vi "(Sub_VI)_CustomPID_BIST.vi"(0 "Process Value":dbl=0.0005 format="%_9g", 1 "Max Out":dbl=0.0005, 2 "Ed_in":dbl, 3 "Min Out":dbl=0.0005, 5 "Set Point":dbl=0.0005 format="%_9g", 7 "Ei_in":dbl, 9 "Kp":dbl, 11 "Kd":dbl, 12 "Ki":dbl) -> (4 "DutyCycle":dbl, 6 "Cp":dbl, 8 "Ei_out":dbl, 10 "Ci":dbl, 13 "Ed_out":dbl, 15 "Cd":dbl)   [LabVIEW 2019]
doc: "The initial value of shift registers (1) and (2) should be left open. If we add zero inside this sub-vi then the integral and the dirivitive of the error is calculated wrong"
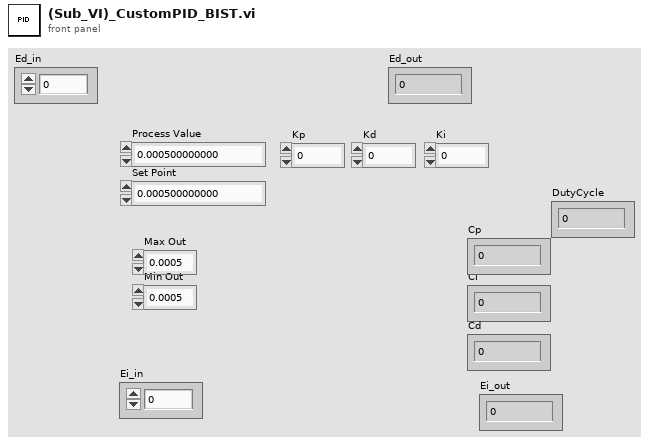
[diagram p1: front panel]
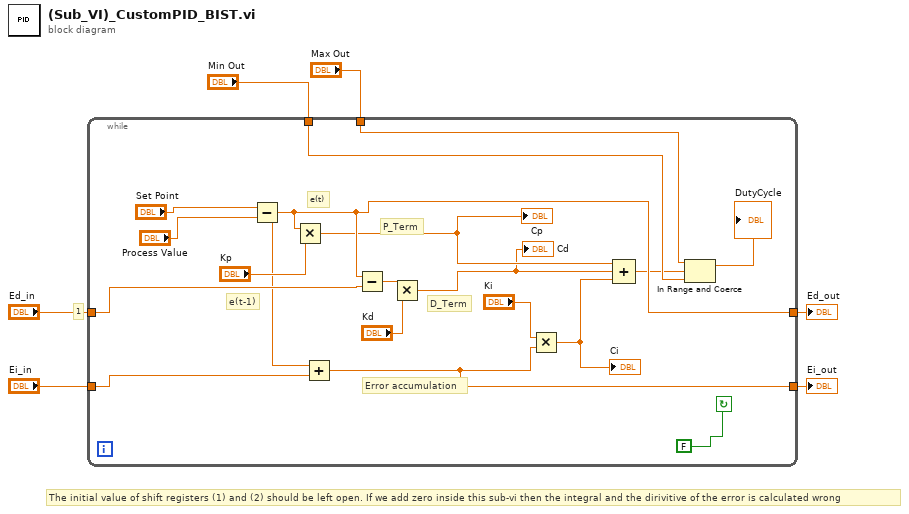
[diagram p0: block diagram]
diagram:
  # "1"
  # "The initial value of shift registers (1) and (2) should be left open. If we add zero inside this sub-vi then the integral and the dirivitive of the error is calculated wrong"
  n1 = while {
    tunnel: "Min Out" -> [w15]
    tunnel: "Max Out" -> [w14]
    tunnel: "Ei_in" -> [w11]
    tunnel: [w17] -> w3
    tunnel: "Ed_in" -> [w21]
    tunnel: [w20] -> w1
    stop <- FALSE ("STOP") continue-if-true
    # "Error accumulation"
    # "D_Term"
    # "P_Term"
    # "e(t-1)"
    # "e(t)"
    n2 = Subtract(x="Set Point", y="Process Value") -> (x-y=w20:dbl)
    n3 = Multiply(x=w20, y="Kp") -> (x*y=w8:dbl)
    "Cp" <- w8
    n4 = Add(x=w20, y=w11) -> (x+y=w17:dbl)
    n5 = Subtract(x=w20, y=w21) -> (x-y=w22:dbl)
    n6 = Multiply(x=w22, y="Kd") -> (x*y=w7:dbl)
    "Cd" <- w7
    n7 = Multiply(x="Ki", y=w17) -> (x*y=w18:dbl)
    "Ci" <- w18
    n8 = Compound Arithmetic op=ADD(w8, w7, w18) -> (w13:dbl)
    n9 = In Range and Coerce(upper limit=w14, x=w13, lower limit=w15) -> (coerced(x)=→"DutyCycle":dbl)  [unwired: 1 out]
  }
  "Ei_out" <- w3
  "Ed_out" <- w1
